vi "Events_Example.vi"() -> ()   [LabVIEW 2018, in "LcWebView.lvclass"]
uses:
  LcWebView.lvclass
  C:/Program Files/National Instruments/LabVIEW 2020/user.lib/_LabVIEWCommon/LcWebView/LcWebView_class/data/Microsoft.Web.WebView2.WinForms.dll
panel:
  in  "Webview container":refnum<k24>(container)
  out "String":string
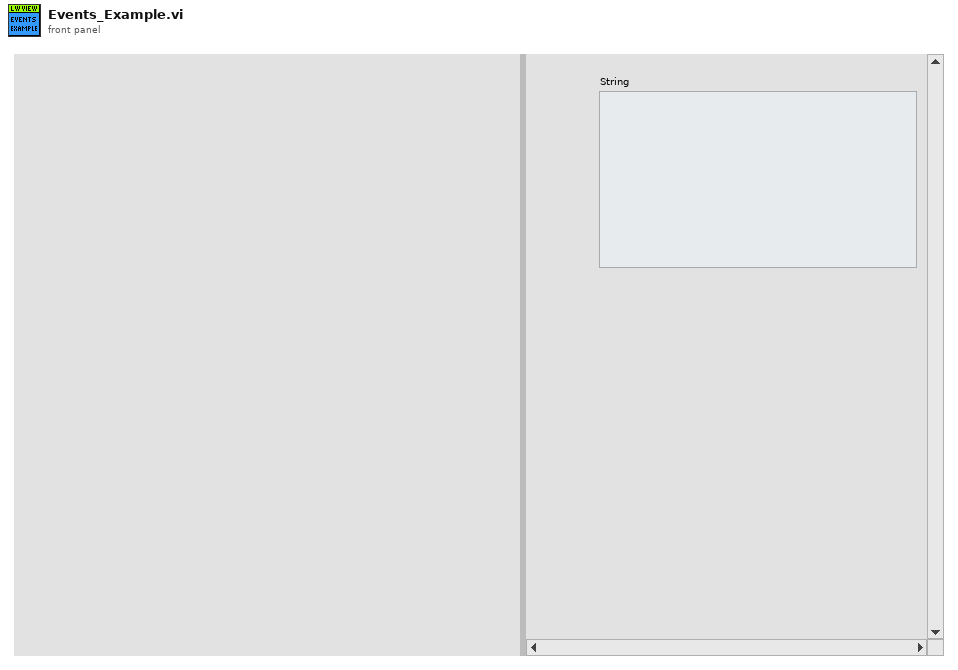
[diagram p1: front panel]
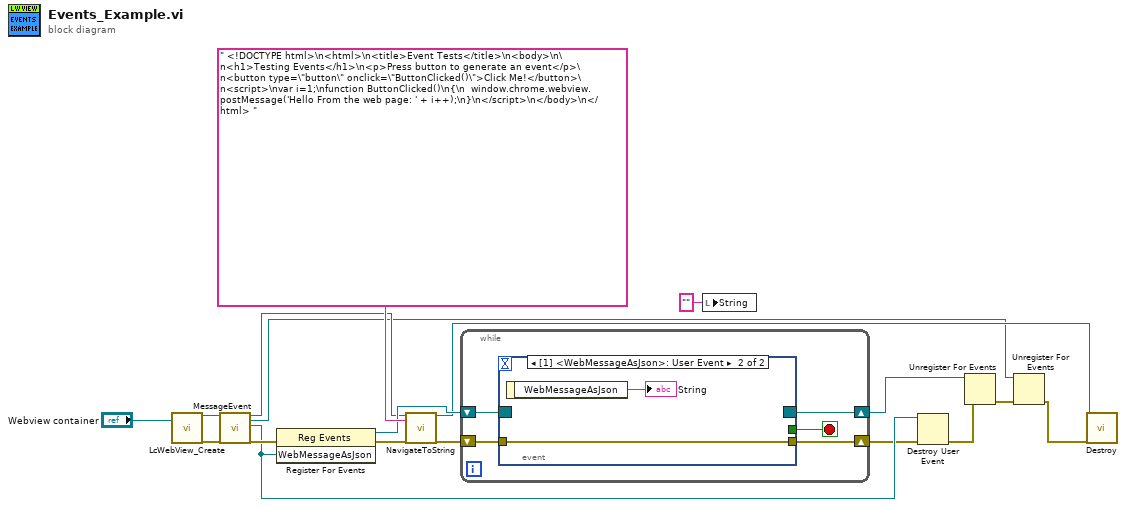
[diagram p0: block diagram]
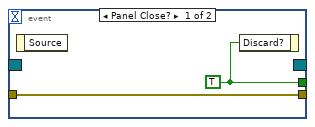
[diagram p2: hidden frame]
diagram:
  n1 = call "LcWebView_Create.vi"("Webview container"="Webview container") -> ("reference out"=w9:refnum<class "LcWebView.lvclass">, "Error Out"=w11:errorcluster)  [unwired: 11 in, 6 out]
  n2 = call "MessageEvent.vi"("reference in"=w9, "error in (no error)"=w11) -> ("reference out"=w8:refnum<class "LcWebView.lvclass">, "Event Callback"=w1:refnum<k27>, "WebMessageAsJson"=w4:refnum<user-event>, "error out"=w13:errorcluster)  [unwired: 14 in]
  n3 = register-events(error in=w13, w4) -> (reference out=w16:refnum<event-registration>, error out=w12:errorcluster)  [unwired: 1 in]
  n4 = call-dynamic "NavigateToString.vi"("reference in"=w8, "HTML Content"=" <!DOCTYPE html>\n<html>\n<title>Event Tests</title>\n<body>\n\n<h1>Testing Events</h1>\n<p>Press button to generate an event</p>\n<button type=\"button\" onclick=\"ButtonClicked()\">Click Me!</button>\n<script>\nvar i=1;\nfunction ButtonClicked()\n{\n  window.chrome.webview.postMessage('Hello From the web page: ' + i++);\n}\n</script>\n</body>\n</html> ", "Error In"=w12) -> ("reference out"=w5:refnum<class "LcWebView.lvclass">, "Error Out"=w10:errorcluster)  [unwired: 14 in, 1 out]
  n5 = while {
    shift-right: [w23] -> w3
    shift-left: w10 -> [w22]
    shift-right: [w20] -> w15
    shift-left: w16 -> [w21]
    stop <- w19 stop-if-true
    n6 = event shown="[1] <WebMessageAsJson>: User Event" {
      selector: w21 -> [_ _]
      dyn-events: [_ _] -> w20
      timeout: _ -> [_ _]
      tunnel: [w25 _] -> w19
      tunnel: w22 -> [w24 w26]
      tunnel: [w24 w26] -> w23
      event Panel Close? {
        w25 = TRUE ("Discard?")
        n7 = event-data() -> ()  [unwired: 1 in, 1 out]
        n8 = event-data("Discard?"=w25) -> ()  [unwired: 1 in, 1 out]
      }
      event User Event {
        n9 = event-data() -> ("WebMessageAsJson"=→"String":string)  [unwired: 1 in]
      }
    }
  }
  n10 = local write "String"("" ("String")) -> ()
  n11 = Destroy User Event(user event=w4, error in=w3) -> (error out=w2:errorcluster)
  n12 = Unregister For Events(event registration refnum=w15, error in=w2) -> (error out=w14:errorcluster)
  n13 = Unregister For Events(event registration refnum=w1, error in=w14) -> (error out=w6:errorcluster)
  n14 = call-dynamic "Destroy.vi"("reference in"=w5, "Error In"=w6) -> ()  [unwired: 16 in, 2 out]
